vi "Clear.vi"(3 "(Index_Pointer) in":refnum<class "Index_Pointer.lvclass">) -> (1 "(Index_Pointer) out":refnum<class "Index_Pointer.lvclass">)   [LabVIEW 2025, in "Index_Pointer.lvclass"]
uses:
  Index_Pointer.lvclass
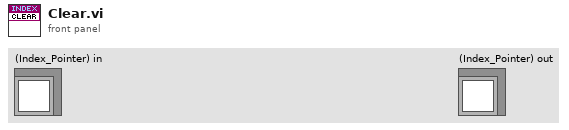
[diagram p1: front panel]
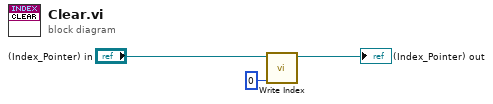
[diagram p0: block diagram]
diagram:
  n1 = call "Write Index.vi"("Index"=0, "(Index_Pointer) In"="(Index_Pointer) in") -> ("(Index_Pointer) Out"=→"(Index_Pointer) out":refnum<class "Index_Pointer.lvclass">)  [unwired: 9 in]
